vi "Files.Rename with Prefix_Count.vi"(8 "error in":errorcluster, 10 "Prefix":string, 11 "Folder":path) -> (0 "error out":errorcluster)   [LabVIEW 2024, in "EQMF.lvlib" / "File Utils.lvlib"]
uses:
  File Utils.lvlib
panel:
  in  "Start":i32=1
  in  "Min Length":i32=3
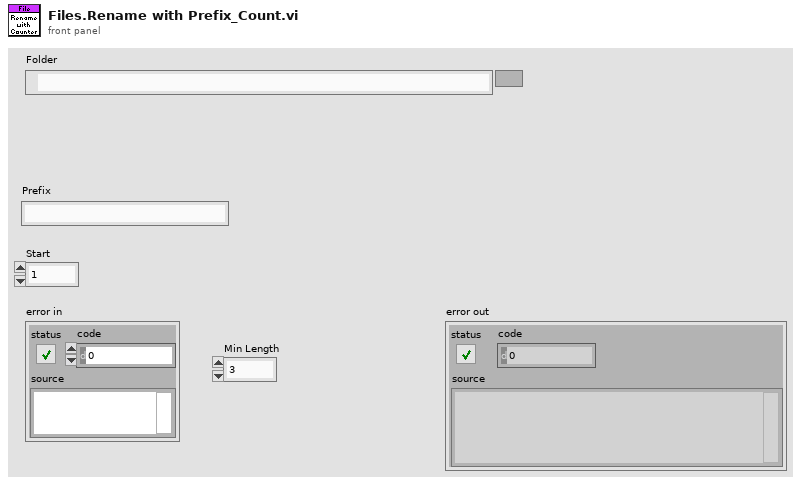
[diagram p1: front panel]
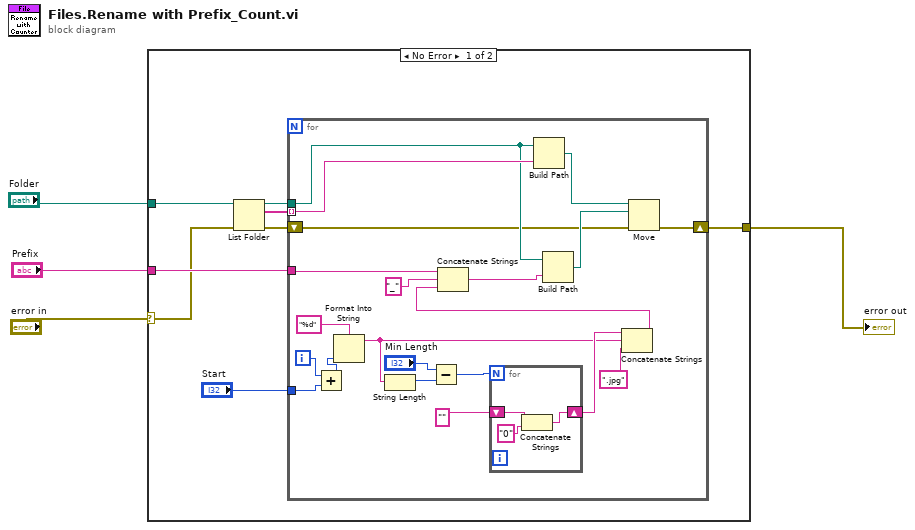
[diagram p0: block diagram]
diagram:
  n1 = case shown="No Error" "error in" {
    selector: "error in" -> [w6 w37]
    tunnel: "Folder" -> [w12 _]
    tunnel: "Prefix" -> [w9 _]
    tunnel: [w7 w37] -> w2
    frame No Error {
      n2 = List Folder(path=w12, error in=w6) -> (path out=w11:path, filenames=w10:string[], error out=w8:errorcluster)  [unwired: 2 in, 1 out]
      n3 = for {
        tunnel: w11 -> [w30]
        tunnel: w10 -> [w33] mode=indexing
        tunnel: w9 -> [w21]
        shift-right: [w28] -> w7
        shift-left: w8 -> [w27]
        tunnel: "Start" -> [w14]
        i -> [w15]
        n4 = Add(x=w15, y=w14) -> (x+y=w13:i32)
        n5 = Format Into String(format string="%d", w13) -> (resulting string=w17:string)  [unwired: 2 in, 1 out]
        n6 = String Length(string=w17) -> (length=w25:i32)
        n7 = Subtract(x="Min Length", y=w25) -> (x-y=w23:i32)
        n8 = for {
          N: w23 -> [_]
          shift-right: [w36] -> w22
          shift-left: "" -> [w35]
          n9 = Concatenate Strings(w35, "0") -> (w36:string)
        }
        n10 = Build Path(base path=w30, name or relative path=w33) -> (appended path=w31:path)
        n11 = Concatenate Strings(w22, w17, ".jpg" ("string")) -> (w19:string)
        n12 = Concatenate Strings(w21, "_", w19) -> (w18:string)
        n13 = Build Path(base path=w30, name or relative path=w18) -> (appended path=w29:path)
        n14 = Move(source path=w31, error in=w27, 10:w29) -> (error out=w28:errorcluster)  [unwired: 2 in, 2 out]
      }
    }
    frame Error {
    }
  }
  "error out" <- w2
